vi "Update GU Test Count And Result.vi"(8 "error in":errorcluster, 10 "Site Data In":T1[](array[typedef]), 11 "Runtime Data In":T3) -> (0 "error out":errorcluster, 1 "Site Data Out":T1[](array[typedef]), 2 "Sites Without Testing":i32[](array[numeric]), 3 "Runtime Data Out":T3)   [LabVIEW 2020, in "GUCalibration2.lvlib"]
uses:
  GUCalibration2.lvlib
  Controls/Config Data Type.ctl
  Controls/Site Data Element.ctl
  Controls/Site Raw Data Element.ctl
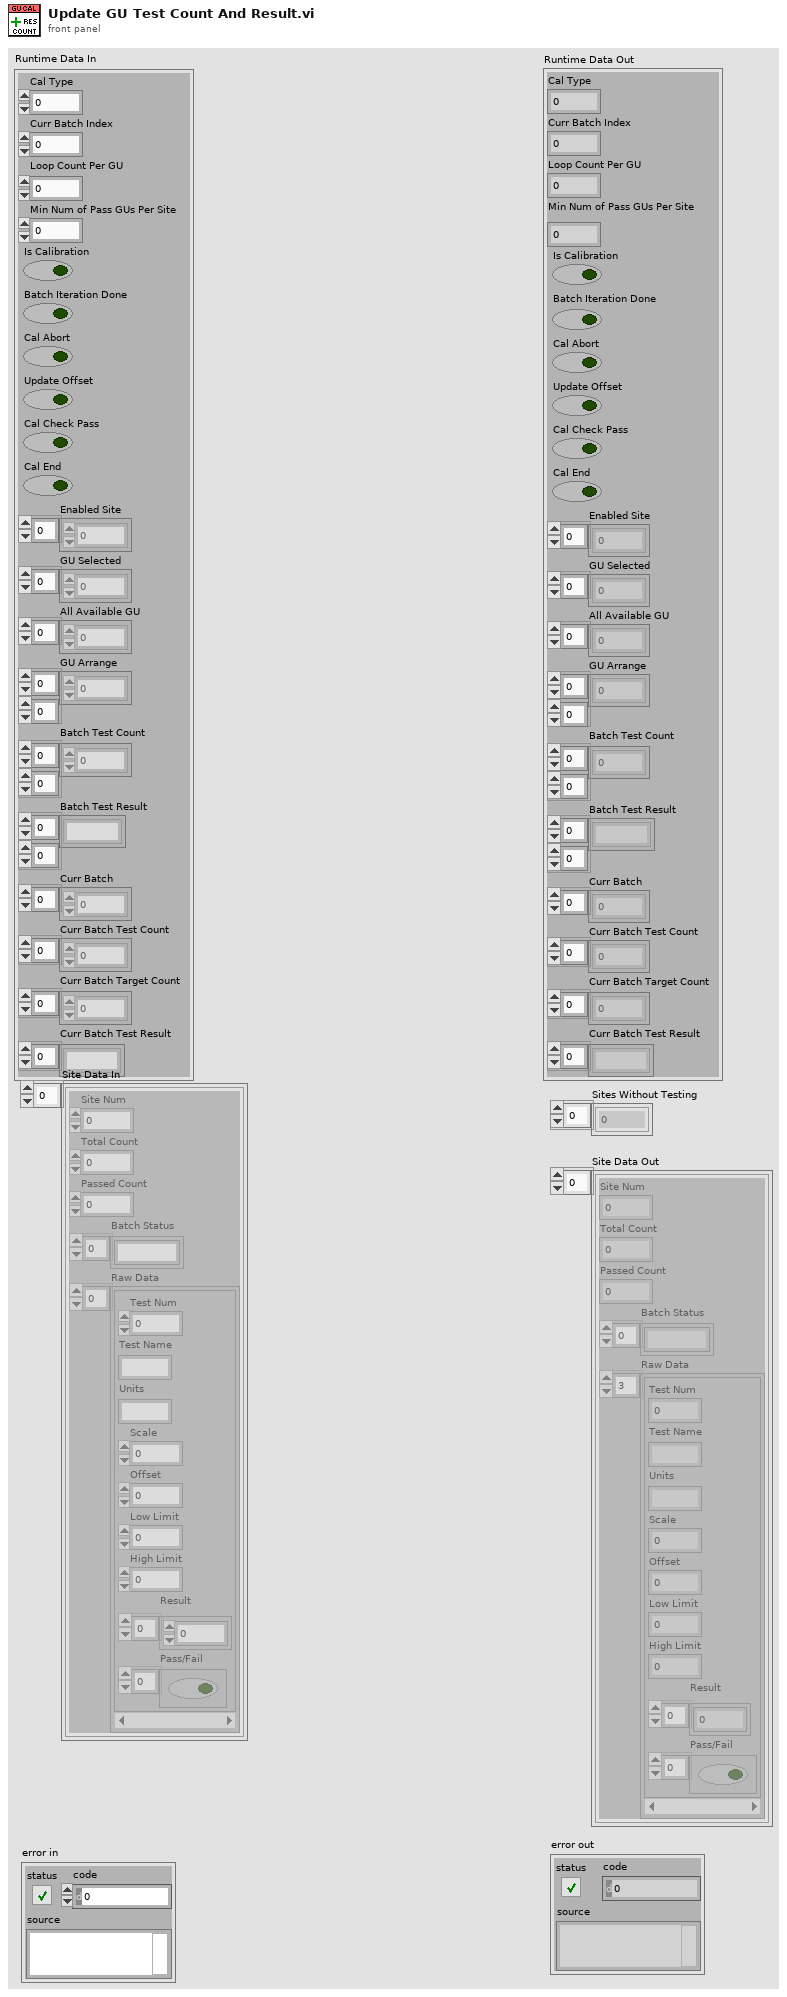
[diagram p1: front panel]
types:
  T1 = typedef "GUCalibration2.lvlib/Site Data Element.ctl" = cluster{"Site Num":i32, "Total Count":i32, "Passed Count":i32, "Batch Status":string[], "Raw Data":T2[]}
  T2 = typedef "GUCalibration2.lvlib/Site Raw Data Element.ctl" = cluster{"Test Num":u32, "Test Name":string, "Units":string, "Scale":i8, "Offset":dbl, "Low Limit":dbl, "High Limit":dbl, "Result":dbl[], "Pass/Fail":bool[]}
  T3 = typedef "GUCalibration2.lvlib/Config Data Type.ctl" = cluster{"Cal Type":i32, "Curr Batch Index":i32, "Loop Count Per GU":i32, "Min Num of Pass GUs Per Site":i32, "Is Calibration":bool, "Batch Iteration Done":bool, "Cal Abort":bool, "Update Offset":bool, "Cal Check Pass":bool, "Cal End":bool, "Enabled Site":i32[], "GU Selected":i32[], "All Available GU":i32[], "GU Arrange":i32[][], "Batch Test Count":i32[][], "Batch Test Result":string[][], "Curr Batch":i32[], "Curr Batch Test Count":i32[], "Curr Batch Target Count":i32[], "Curr Batch Test Result":string[]}
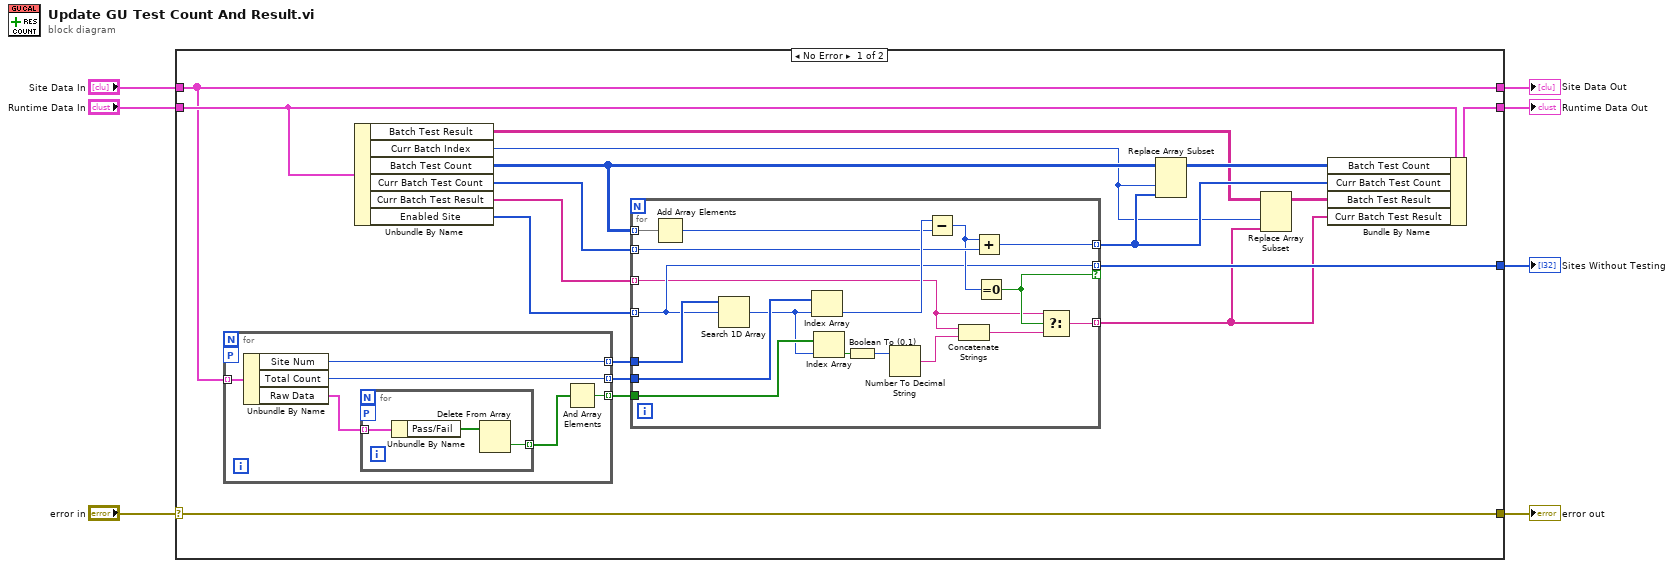
[diagram p0: block diagram]
diagram:
  n1 = case shown="No Error" "error in" {
    selector: "error in" -> [w9 w53]
    tunnel: "Runtime Data In" -> [w22 w55]
    tunnel: [w21 w55] -> w6
    tunnel: [w20 _] -> w5
    tunnel: [w9 w53] -> w3
    tunnel: "Site Data In" -> [w8 w54]
    tunnel: [w8 w54] -> w1
    frame No Error {
      n2 = for {
        tunnel: w8 -> [w49] mode=indexing
        tunnel: [w48] -> w25 mode=indexing
        tunnel: [w47] -> w24 mode=indexing
        tunnel: [w44] -> w23 mode=indexing
        workers-P: _ -> [_]
        n3 = Unbundle By Name(w49) -> ("Site Num"=w48:i32, "Total Count"=w47:i32, "Raw Data"=w46:T2[])
        n4 = for {
          tunnel: w46 -> [w52] mode=indexing
          tunnel: [w50] -> w45 mode=indexing
          workers-P: _ -> [_]
          n5 = Unbundle By Name(w52) -> ("Pass/Fail"=w51:bool[])
          n6 = Delete From Array(array=w51) -> (deleted portion=w50:bool)  [unwired: 2 in, 1 out]
        }
        n7 = And Array Elements(Boolean array=w45) -> (logical AND=w44:bool)
      }
      n8 = Unbundle By Name(w22) -> ("Batch Test Result"=w13:string[][], "Curr Batch Index"=w12:i32, "Batch Test Count"=w19:i32[][], "Curr Batch Test Count"=w16:i32[], "Curr Batch Test Result"=w14:string[], "Enabled Site"=w15:i32[])
      n9 = for {
        tunnel: w15 -> [w33] mode=indexing
        tunnel: w25 -> [w43]
        tunnel: w24 -> [w42]
        tunnel: w23 -> [w41]
        tunnel: w19 -> [w39] mode=indexing
        tunnel: w16 -> [w36] mode=indexing
        tunnel: [w35] -> w18 mode=indexing
        tunnel: [w33] -> w20 mode=indexing if=w29
        tunnel: w14 -> [w27] mode=indexing
        tunnel: [w26] -> w10 mode=indexing
        n10 = Add Array Elements(numeric array=w39) -> (sum=w37:i32)
        n11 = Search 1D Array(1D array=w43, element=w33) -> (index of element=w40:i32)  [unwired: 1 in]
        n12 = Index Array(array=w42, index=w40) -> (element=w38:i32)
        n13 = Index Array(array=w41, index=w40) -> (element=w32:bool)
        n14 = Boolean To (0,1)(Boolean=w32) -> (0, 1=w31:i16)
        n15 = Number To Decimal String(number=w31) -> (decimal integer string=w30:string)  [unwired: 1 in]
        n16 = Subtract(x=w38, y=w37) -> (x-y=w34:i32)
        n17 = Concatenate Strings(w27, w30) -> (w28:string)
        n18 = Add(x=w34, y=w36) -> (x+y=w35:i32)
        n19 = Equal To 0?(x=w34) -> (x = 0?=w29:bool)
        n20 = Select(t=w27, s=w29, f=w28) -> (s? t:f=w26:string)
      }
      n21 = Replace Array Subset(array=w19, new element=w18, index (col)=w12) -> (w17:i32[][])  [unwired: 1 in]
      n22 = Replace Array Subset(array=w13, new element=w10, index (col)=w12) -> (w11:string[][])  [unwired: 1 in]
      n23 = Bundle By Name(cluster=w22, "Batch Test Count"=w17, "Curr Batch Test Count"=w18, "Batch Test Result"=w11, "Curr Batch Test Result"=w10) -> (w21:T3)
    }
    frame Error {
    }
  }
  "Runtime Data Out" <- w6
  "Sites Without Testing" <- w5
  "error out" <- w3
  "Site Data Out" <- w1
